vi "Publish and Subscribe Queue-based.vi"() -> ()   [LabVIEW 2020, in "wamplv.lvlib"]
uses:
  <vilib>/samangh/wamplv/WAMP Client/TypeDef/wamplv.lvlib
  <vilib>/samangh/wamplv/WAMP Client/API/New WebSocket Client.vi
  <vilib>/samangh/wamplv/WAMP Client/WAMP Client.lvclass
panel:
  in  "Unregister RPC":bool caption="Publish Topic"
  in  "Endpoint return value":string="test.topic"
  in  "Register RPC":bool caption="Publish Topic"
  out "Error URI":string
  out "Callee Error?":bool
  out "Call Result ArgumentKw":string
  out "Call Result Arguments":string[](array[string])
  in  "Call Arguments":string[](array[string])
  in  "Call URI":string="test.endpoint"
  in  "Call":bool caption="Publish Topic"
  in  "Unsubscribe":bool caption="Publish Topic"
  out "Topic:":string
  out "ArgumentKw Payload":string
  out "Arguments Payload":string[](array[string])
  out "Event received on:":string
  in  "Publish Argument Payload":string[](array[string])
  in  "Subscription URI":string="test.topic"
  in  "Subscribe":bool caption="Publish Topic"
  in  "Disconnect":bool caption="Publish Topic"
  in  "Realm":string="default_realm"
  in  "Topic URI":string="test.topic"
  in  "Publish":bool caption="Publish Topic"
  in  "Router Address":string="ws://localhost:8080/"
  # "Endpoint name: test.endpoint"
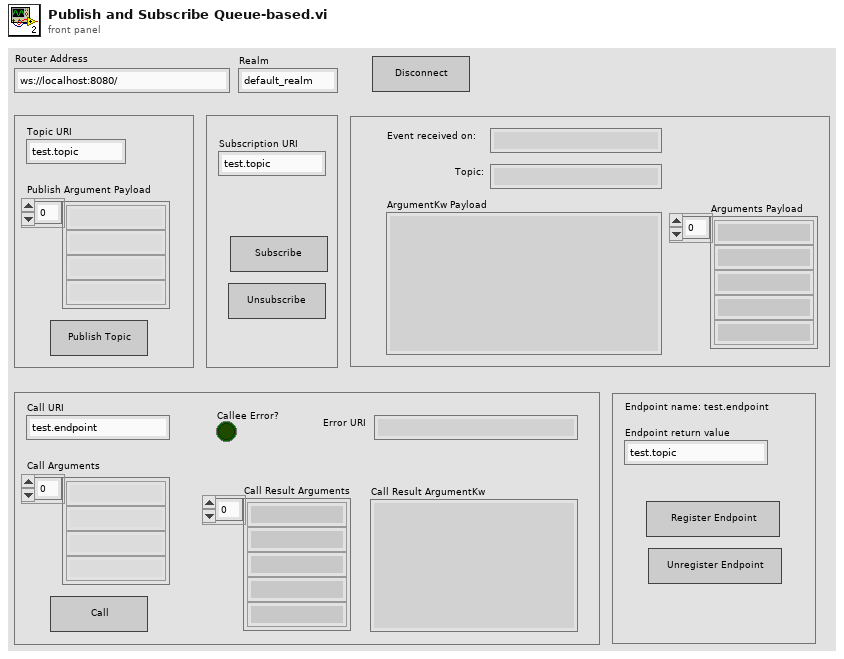
[diagram p1: front panel]
types:
  T1 = typedef "wamplv.lvlib/WAMP Client.lvclass/WAMP Error Payload.ctl" = cluster{"Details":string, "ArgumentKw Payload":string, "Wamp error?":bool, "Error URI":string, "Arguments Payload":string[]}
  T2 = typedef "wamplv.lvlib/WAMP Client.lvclass/INVOCATION payload.ctl" = cluster{"Arguments":string[], "ArgumentKw":string, "Procedure URI":string, "Details":string, "Registration ID":u64, "Request ID":u64}
  T3 = typedef "wamplv.lvlib/WAMP Client.lvclass/Event Payload.ctl" = cluster{"Arguments Payload":string[], "ArgumentKw Payload":string, "Topic":string}
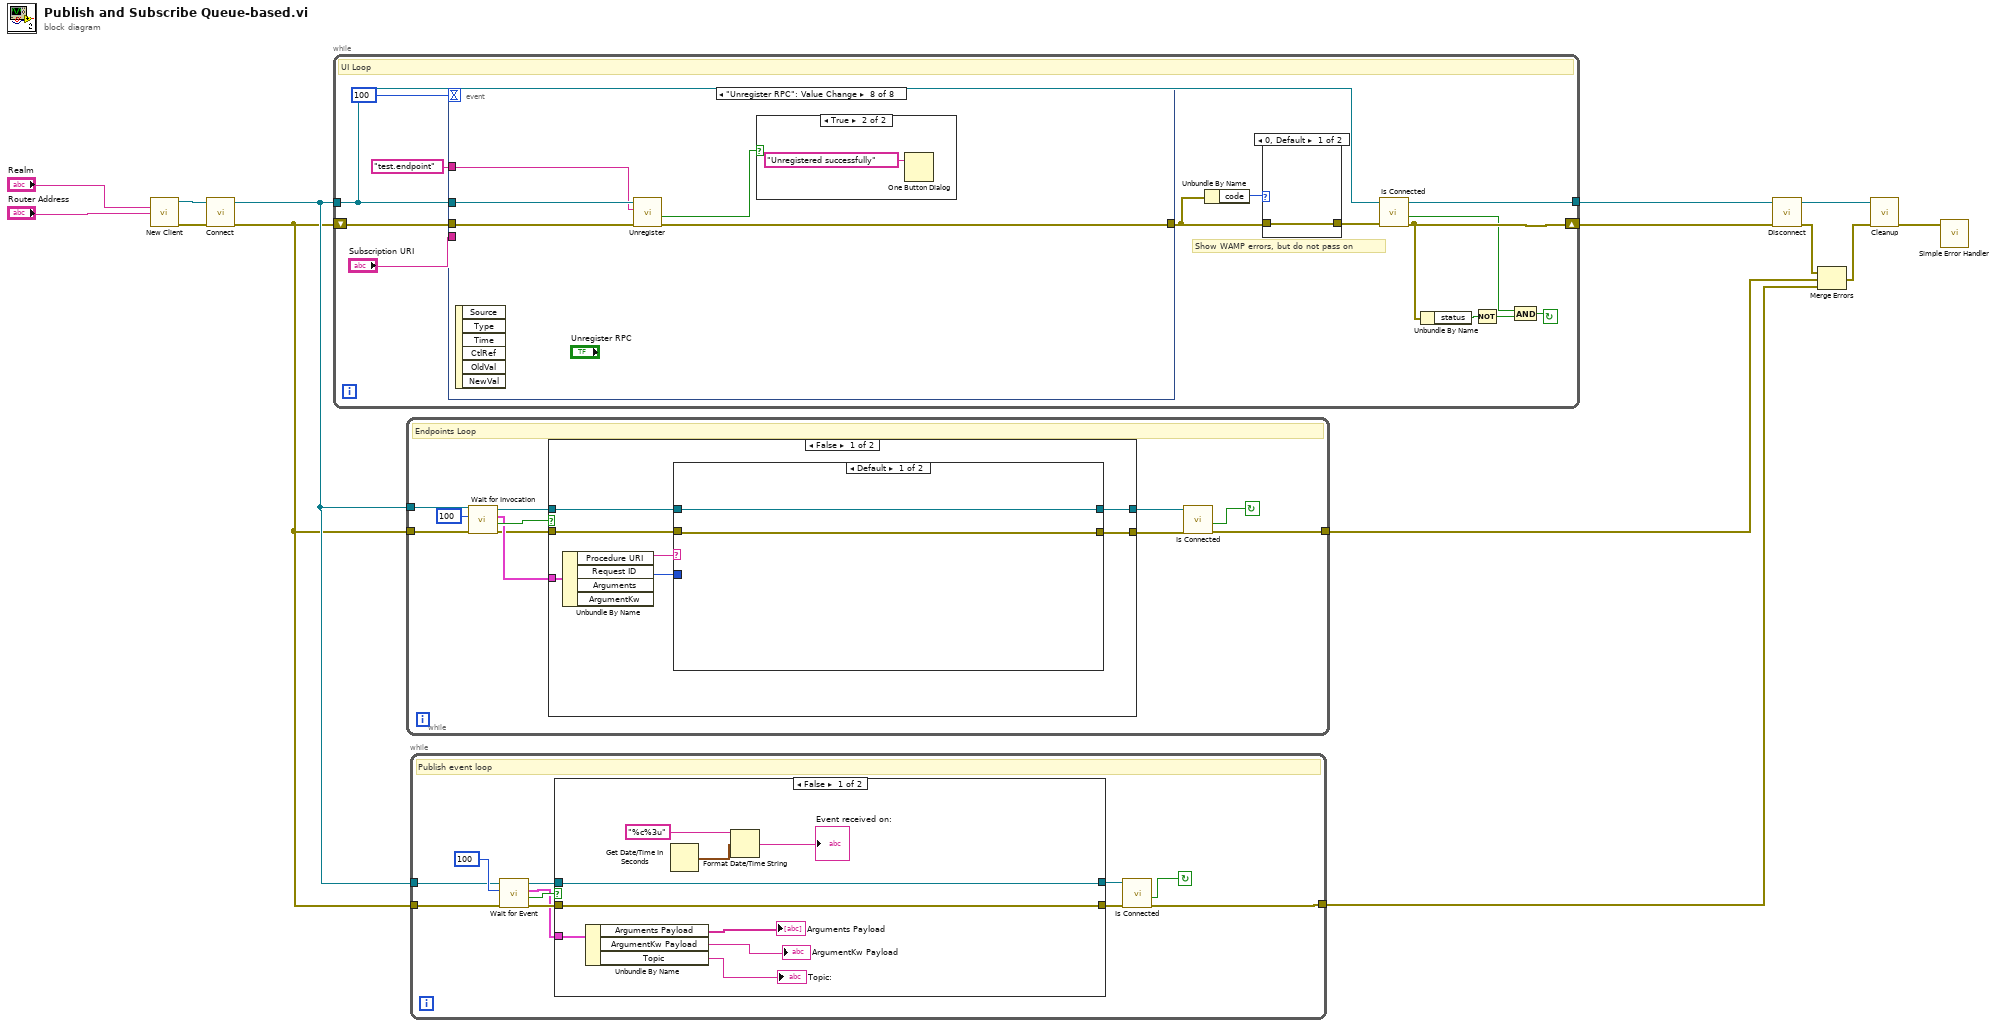
[diagram p0: block diagram]
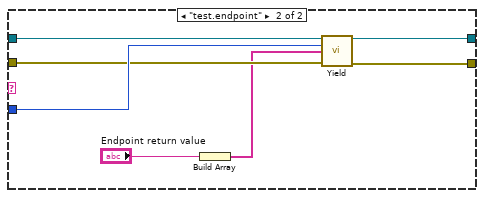
[diagram p3: hidden frame]
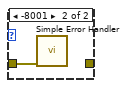
[diagram p5: hidden frame]
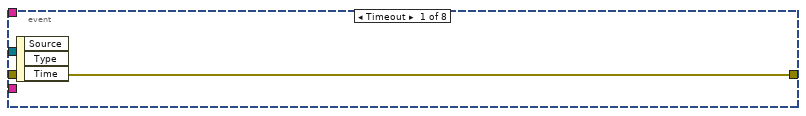
[diagram p6: hidden frame]
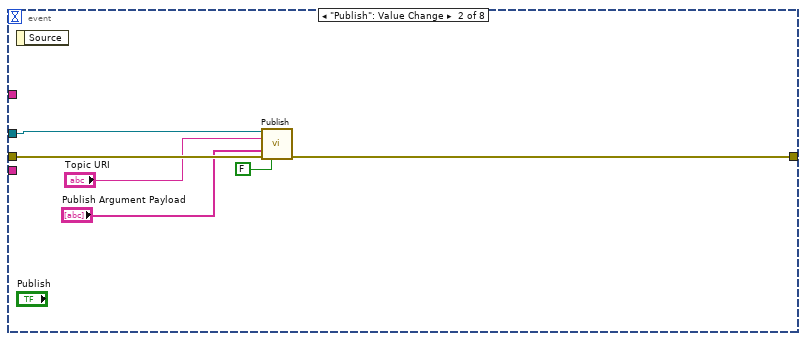
[diagram p7: hidden frame]
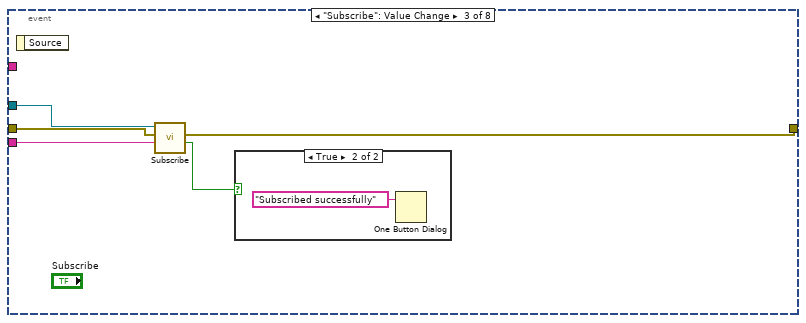
[diagram p8: hidden frame]
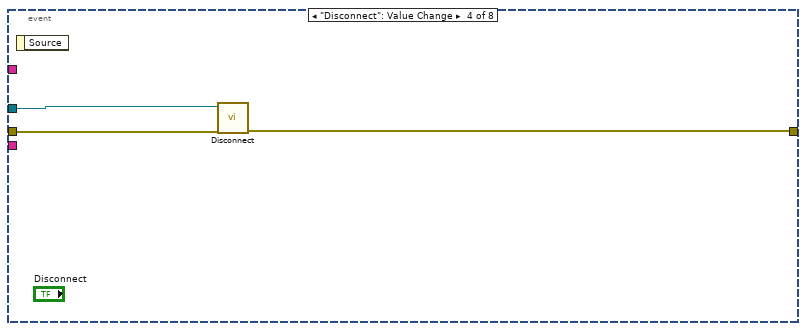
[diagram p10: hidden frame]
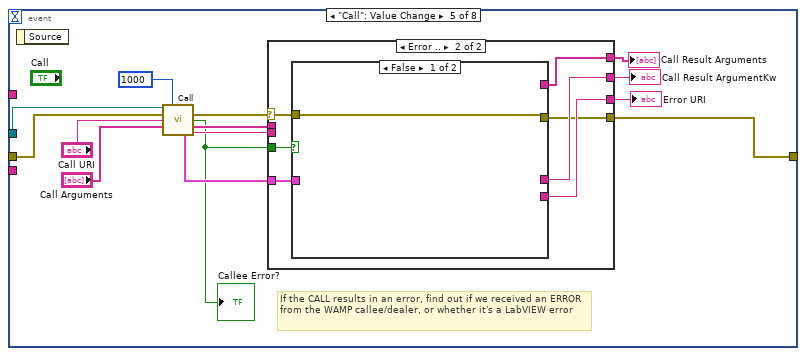
[diagram p11: hidden frame]
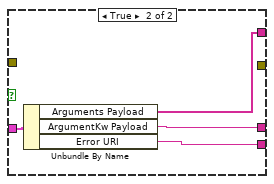
[diagram p13: hidden frame]
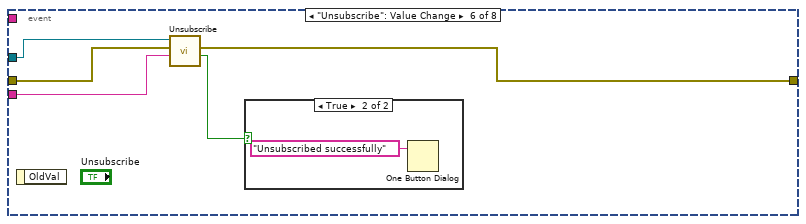
[diagram p14: hidden frame]
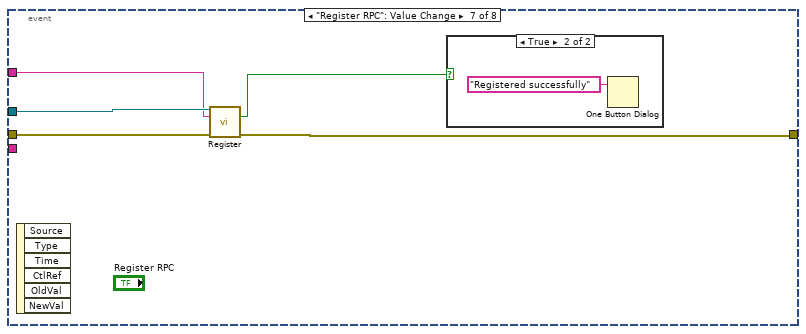
[diagram p16: hidden frame]
diagram:
  n1 = call-poly <vilib>:"New Client.vi"("Realm"="Realm", "Address"="Router Address") -> ("reference out"=w12:refnum<class "WAMP Client.lvclass">, "error out"=w4:errorcluster)  [unwired: 12 in]
  n2 = call <vilib>:"Connect.vi"("error in (no error)"=w4, "WAMP Client in"=w12) -> ("error out"=w3:errorcluster, "WAMP Client out"=w6:refnum<class "WAMP Client.lvclass">)  [unwired: 8 in]
  n3 = while {
    tunnel: w6 -> [w26]
    shift-right: [w18] -> w2
    shift-left: w3 -> [w28]
    tunnel: [w25] -> w5
    stop <- w19 continue-if-true
    # "Show WAMP errors, but do not pass on"
    # "UI Loop"
    n4 = event shown="[7] \"Unregister RPC\": Value Change" {
      selector: _ -> [_ _ _ _ _ _ _ _]
      dyn-events: _ -> [_ _ _ _ _ _ _ _]
      timeout: 100 -> [_ _ _ _ _ _ _ _]
      tunnel: w26 -> [_ w37 w42 w46 w60 w79 w86 w92]
      tunnel: w28 -> [w31 w36 w41 w45 w59 w80 w85 w91]
      tunnel: [w31 w35 w40 w44 w56 w78 w84 w89] -> w21
      tunnel: "Subscription URI" -> [_ _ w38 _ _ w76 _ _]
      tunnel: "test.endpoint" ("Procedure URI") -> [_ _ _ _ _ _ w83 w90]
      event Timeout {
        n5 = event-data() -> ()  [unwired: 1 in, 3 out]
      }
      event "Publish": Value Change {
        n6 = event-data() -> ()  [unwired: 1 in, 1 out]
        n7 = call-dynamic "Publish.vi"("WAMP Client in"=w37, "Topic"="Topic URI", "Arguments"="Publish Argument Payload", "error in (no error)"=w36, "Request Ack."=FALSE) -> ("error out"=w35:errorcluster)  [unwired: 9 in, 1 out]
      }
      event "Subscribe": Value Change {
        n8 = event-data() -> ()  [unwired: 1 in, 1 out]
        n9 = call-dynamic "Subscribe.vi"("Topic"=w38, "error in (no error)"=w41, "WAMP Client in"=w42) -> ("Success?"=w39:bool, "error out"=w40:errorcluster)  [unwired: 3 in, 2 out]
        n10 = case shown="True" w39 {
          frame False {
          }
          frame True {
            n11 = One Button Dialog(message="Subscribed successfully") -> ()  [unwired: 1 in, 1 out]
          }
        }
      }
      event "Disconnect": Value Change {
        n12 = event-data() -> ()  [unwired: 1 in, 1 out]
        n13 = call-dynamic "Disconnect.vi"("error in (no error)"=w45, "WAMP Client in"=w46) -> ("error out"=w44:errorcluster)  [unwired: 8 in, 1 out]
      }
      event "Call": Value Change {
        # "If the CALL results in an error, find out if we received an ERROR from the WAMP callee/dealer, or whether it's a LabVIEW error"
        n14 = event-data() -> ()  [unwired: 1 in, 1 out]
        n15 = call-dynamic "Call.vi"("WAMP Client in"=w60, "Numeric"=1000, "error in"=w59, "Topic URI"="Call URI", "Arguments"="Call Arguments") -> ("error out"=w57:errorcluster, "WAMP Error?"=w48:bool, "Arguments Payload"=w54:string[], "WAMP Error"=w50:T1, "ArgumentKw Payload"=w53:string)  [unwired: 5 in, 1 out]
        "Callee Error?" <- w48
        n16 = case shown="Error .." w57 {
          selector: w57 -> [w63 w66]
          tunnel: [w63 w65] -> w56
          tunnel: [w62 w64] -> w55
          tunnel: w54 -> [w62 _]
          tunnel: w53 -> [w61 _]
          tunnel: [w61 w68] -> w52
          tunnel: w48 -> [_ w70]
          tunnel: [_ w67] -> w51
          tunnel: w50 -> [_ w69]
          frame No Error {
          }
          frame Error {
            n17 = case shown="False" w70 {
              tunnel: w69 -> [_ w75]
              tunnel: [_ w74] -> w68
              tunnel: [_ w73] -> w67
              tunnel: w66 -> [w71 _]
              tunnel: [w71 _] -> w65
              tunnel: [_ w72] -> w64
              frame False {
              }
              frame True {
                n18 = Unbundle By Name(w75) -> ("Arguments Payload"=w72:string[], "ArgumentKw Payload"=w74:string, "Error URI"=w73:string)
              }
            }
          }
        }
        "Call Result Arguments" <- w55
        "Call Result ArgumentKw" <- w52
        "Error URI" <- w51
      }
      event "Unsubscribe": Value Change {
        n19 = event-data() -> ()  [unwired: 1 in, 1 out]
        n20 = call-dynamic "Unsubscribe.vi"("Topic"=w76, "error in (no error)"=w80, "WAMP Client in"=w79) -> ("Success?"=w77:bool, "error out"=w78:errorcluster)  [unwired: 4 in, 1 out]
        n21 = case shown="True" w77 {
          frame False {
          }
          frame True {
            n22 = One Button Dialog(message="Unsubscribed successfully") -> ()  [unwired: 1 in, 1 out]
          }
        }
      }
      event "Register RPC": Value Change {
        n23 = event-data() -> ()  [unwired: 1 in, 6 out]
        n24 = call-dynamic "Register.vi"("WAMP Client in"=w86, "Procedure URI"=w83, "error in (no error)"=w85) -> ("Success?"=w82:bool, "error out"=w84:errorcluster)  [unwired: 9 in, 2 out]
        n25 = case shown="True" w82 {
          frame False {
          }
          frame True {
            n26 = One Button Dialog(message="Registered successfully") -> ()  [unwired: 1 in, 1 out]
          }
        }
      }
      event "Unregister RPC": Value Change {
        n27 = event-data() -> ()  [unwired: 1 in, 6 out]
        n28 = call-dynamic "Unregister.vi"("error in (no error)"=w91, "URI"=w90, "WAMP Client in"=w92) -> ("error out"=w89:errorcluster, "Success?"=w88:bool)  [unwired: 4 in, 1 out]
        n29 = case shown="True" w88 {
          frame False {
          }
          frame True {
            n30 = One Button Dialog(message="Unregistered successfully") -> ()  [unwired: 1 in, 1 out]
          }
        }
      }
    }
    n31 = Unbundle By Name(w21) -> ("code"=w22:i32)
    n32 = case shown="0, Default" w22 {
      tunnel: w21 -> [w29 w30]
      tunnel: [w29 _] -> w20
      frame 0, Default {
      }
      frame -8001 {
        n33 = call <vilib>:"Simple Error Handler.vi"("error in (no error)"=w30) -> ()  [unwired: 4 in, 5 out]
      }
    }
    n34 = call-dynamic "Is Connected.vi"("error in (no error)"=w20, "WAMP Client in"=w26) -> ("error out"=w18:errorcluster, "Is Connected?"=w15:bool, "WAMP Client out"=w25:refnum<class "WAMP Client.lvclass">)  [unwired: 7 in]
    n35 = Unbundle By Name(w18) -> ("status"=w17:bool)
    n36 = Not(x=w17) -> (.not. x?=w16:bool)
    n37 = And(x=w15, y=w16) -> (x .and. y?=w19:bool)
  }
  n38 = while {
    tunnel: w6 -> [w104]
    tunnel: w3 -> [w103]
    tunnel: [w94] -> w8
    stop <- w95 continue-if-true
    # "Endpoints Loop"
    n39 = call-dynamic "Wait for Invocation.vi"("error in (no error)"=w103, "timeout in ms (-1)"=100, "WAMP Client in"=w104) -> ("error out"=w98:errorcluster, "timed out?"=w101:bool, "WAMP Invocation"=w99:T2, "WAMP Client out"=w100:refnum<class "WAMP Client.lvclass">)  [unwired: 5 in]
    n40 = case shown="False" w101 {
      tunnel: w100 -> [w109 w122]
      tunnel: w99 -> [w111 _]
      tunnel: w98 -> [w107 w121]
      tunnel: [w106 w121] -> w96
      tunnel: [w105 w122] -> w97
      frame False {
        n41 = Unbundle By Name(w111) -> ("Procedure URI"=w110:string, "Request ID"=w108:u64)  [unwired: 2 out]
        n42 = case shown="Default" w110 {
          tunnel: w109 -> [w113 w120]
          tunnel: w108 -> [_ w119]
          tunnel: w107 -> [w112 w118]
          tunnel: [w112 w117] -> w106
          tunnel: [w113 w116] -> w105
          frame Default {
          }
          frame "test.endpoint" {
            n43 = Build Array("Endpoint return value") -> (w115:string[])
            n44 = call <vilib>:"Yield.vi"("WAMP Client in"=w120, "Invocation Request ID"=w119, "Arguments"=w115, "error in (no error)"=w118) -> ("WAMP Client out"=w116:refnum<class "WAMP Client.lvclass">, "error out"=w117:errorcluster)  [unwired: 10 in]
          }
        }
      }
      frame True {
      }
    }
    n45 = call-dynamic "Is Connected.vi"("error in (no error)"=w96, "WAMP Client in"=w97) -> ("error out"=w94:errorcluster, "Is Connected?"=w95:bool)  [unwired: 7 in, 1 out]
  }
  n46 = while {
    tunnel: w6 -> [w132]
    tunnel: w3 -> [w131]
    tunnel: [w123] -> w7
    stop <- w124 continue-if-true
    # "Publish event loop"
    n47 = call-dynamic "Wait for Event.vi"("error in (no error)"=w131, "timeout in ms (-1)"=100, "WAMP Client in"=w132) -> ("error out"=w128:errorcluster, "timed out?"=w130:bool, "WAMP Event"=w127:T3, "WAMP Client out"=w129:refnum<class "WAMP Client.lvclass">)  [unwired: 5 in]
    n48 = case shown="False" w130 {
      tunnel: w129 -> [w135 w143]
      tunnel: w128 -> [w134 w144]
      tunnel: w127 -> [w139 _]
      tunnel: [w135 w143] -> w126
      tunnel: [w134 w144] -> w125
      frame False {
        n49 = Unbundle By Name(w139) -> ("Arguments Payload"=→"Arguments Payload":string[], "ArgumentKw Payload"=→"ArgumentKw Payload":string, "Topic"=→"Topic:":string)
        n50 = Get Date/Time In Seconds() -> (seconds since 1Jan1904=w141:timestamp)
        n51 = Format Date/Time String(time format string (%c)="%c%3u", seconds (now)=w141) -> (date/time string=→"Event received on:":string)  [unwired: 1 in]
      }
      frame True {
      }
    }
    n52 = call-dynamic "Is Connected.vi"("error in (no error)"=w125, "WAMP Client in"=w126) -> ("error out"=w123:errorcluster, "Is Connected?"=w124:bool)  [unwired: 7 in, 1 out]
  }
  n53 = call-dynamic "Disconnect.vi"("error in (no error)"=w2, "WAMP Client in"=w5) -> ("error out"=w1:errorcluster, "WAMP Client out"=w11:refnum<class "WAMP Client.lvclass">)  [unwired: 8 in]
  n54 = Merge Errors(w1, w8, w7) -> (w10:errorcluster)
  n55 = call-dynamic "Cleanup.vi"("error in (no error)"=w10, "WAMP Client in"=w11) -> ("error out"=w9:errorcluster)  [unwired: 8 in, 1 out]
  n56 = call <vilib>:"Simple Error Handler.vi"("error in (no error)"=w9) -> ()  [unwired: 4 in, 5 out]
